vi "Build_Array.vi"(1 "Ncolumns":i32, 2 "Nrows":i32) -> (0 "Array":dbl[][](array[numeric]))   [LabVIEW 2018]
doc: "Return a zeroed array of a given size\n\nNo. rows = number of data sets\n\nNo. cols = data points in each row\n\nR. Sheehan 5 - 11 - 2016"
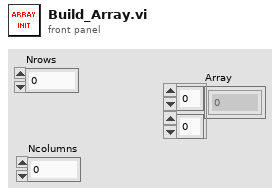
[diagram p1: front panel]
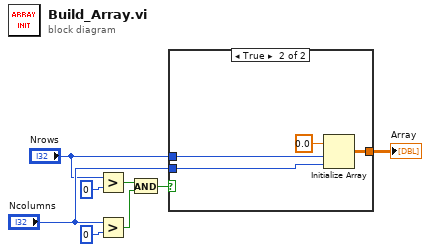
[diagram p0: block diagram]
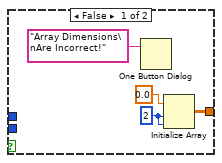
[diagram p2: hidden frame]
diagram:
  n1 = Greater?(x="Nrows", y=0) -> (0:w6:bool)
  n2 = Greater?(x="Ncolumns", y=0) -> (0:w5:bool)
  n3 = And(x=w6, y=w5) -> (x .and. y?=w4:bool)
  n4 = case shown="True" w4 {
    tunnel: "Ncolumns" -> [_ w15]
    tunnel: "Nrows" -> [_ w14]
    tunnel: [w9 w13] -> w1
    frame False {
      w10 = 2 ("dimension size")
      n5 = One Button Dialog(message="Array Dimensions\nAre Incorrect!") -> ()  [unwired: 1 in, 1 out]
      n6 = Initialize Array(0.0 ("element"), w10, w10) -> (w9:dbl[][])
    }
    frame True {
      n7 = Initialize Array(0.0 ("element"), w14, w15) -> (w13:dbl[][])
    }
  }
  "Array" <- w1
